vi "Override Error.vi"(10 "Error":errorcluster, 11 "jettl Event Actor in":refnum<class "jettl Event Actor.lvclass">) -> (3 "jettl Event Actor out":refnum<class "jettl Event Actor.lvclass">)   [LabVIEW 2021, in "jettl.lvlib" / "jettl Event Actor.lvclass"]
uses:
  jettl Event Actor.lvclass
  jettl Event Actor.lvclass/jettl Event Actor.ctl
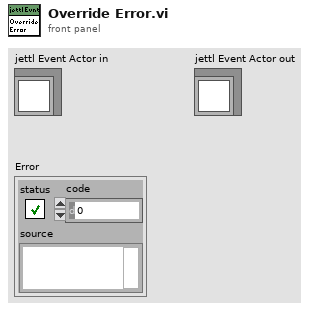
[diagram p1: front panel]
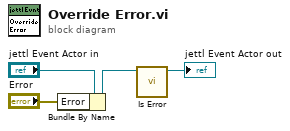
[diagram p0: block diagram]
diagram:
  n1 = Bundle By Name(cluster="jettl Event Actor in", "Error"="Error") -> (w2:refnum<class "jettl Event Actor.lvclass">)
  n2 = call "Is Error.vi"("jettl Event Actor in"=w2) -> ("jettl Event Actor out"=→"jettl Event Actor out":refnum<class "jettl Event Actor.lvclass">)  [unwired: 10 in]
